vi "Send Results to UI.vi"(8 "error in (no error)":errorcluster, 10 "Results.lvclass":refnum<class "Results.lvclass">, 11 "UI Queue":refnum<class "Message Enqueuer.lvclass">) -> (0 "error out":errorcluster, 3 "UI Queue Out":refnum<class "Message Enqueuer.lvclass">)   [LabVIEW 2016, in "Controller UI.lvlib" / "Display Results.lvclass"]
uses:
  <userlib>/Common Components/User Interface/Messages/Display Results/Display Results.lvclass
  <userlib>/Common Components/Results/Results.lvclass
  <vilib>/ActorFramework/Message Enqueuer/Message Enqueuer.lvclass
  C:/Program Files (x86)/National Instruments/LabVIEW 2016/vi.lib/ActorFramework/Message/Message.lvclass
  <vilib>/ActorFramework/Message Enqueuer/Message Enqueuer.lvclass/Message Enqueuer.ctl
  <vilib>/ActorFramework/Message Priority Queue/Priority Enqueue.vi
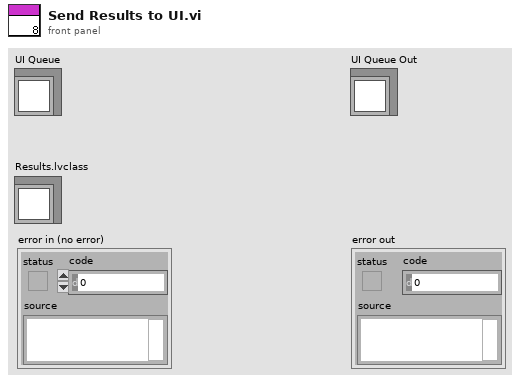
[diagram p1: front panel]
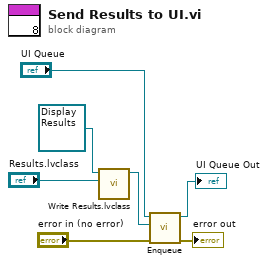
[diagram p0: block diagram]
diagram:
  n1 = call <userlib>:"Write Results.lvclass.vi"("Results.lvclass"="Results.lvclass", "Display Results in"=refnum<class "Display Results.lvclass"> refnum ("Display Results.lvclass")) -> ("Display Results out"=w3:refnum<class "Display Results.lvclass">)  [unwired: 8 in, 1 out]
  n2 = call <vilib>:"Enqueue.vi"("error in (no error)"="error in (no error)", "Message"=w3, "Message Enqueuer in"="UI Queue") -> ("error out"=→"error out":errorcluster, "Message Enqueuer out"=→"UI Queue Out":refnum<class "Message Enqueuer.lvclass">)  [unwired: 7 in]
